vi "StitchAxialZones.vi"(4 "z increment axial":dbl=0.125, 5 "FileStartName":string, 6 "pressures in":dbl[][][](array[numeric]), 7 "Scales":dbl[](array[numeric]), 8 "z increment":dbl=0.125, 9 "z Start pos":sgl=7.0) -> (0 "6dB data":dbl[][](array[numeric]), 1 "Focal zones joined":dbl[][](array[numeric]), 2 "Axial Beam":cluster{sgl, dbl, sgl[]}(graph), 3 "lateral segs":cluster{dbl, dbl, dbl[][]}(graph))   [LabVIEW 2022 SP3]
uses:
  <vilib>/Math Plots/3D Math Plots/3D Surface/3D Surface XCtrl/3D Surface.xctl
  <vilib>/Math Plots/3D Math Plots/3D Surface/3D Surface Datatype/Public/Plot Helper (Vector).vi
  <vilib>/Utility/file.llb/Write Delimited Spreadsheet (DBL).vi
  <vilib>/Math Plots/3D Math Plots/3D Surface/3D Surface Datatype/3D Surface Datatype.lvclass
panel:
  in  "Tab Control":enum32{"Page 1", "Page 2"}(tab)
  out "Lateral 6dB":cluster{dbl[], dbl[]}(graph)
  out "Axia focal zone stitch":cluster{dbl[], dbl[]}(graph)
  in  "Save lateal profiles":bool
  in  "Save lateal BWs":bool
  in  "Save axial profile":bool
  out "3D Surface":refnum<class "3D Plot Datatype.lvclass">[](xcontrol)
  out "axial segs":cluster{sgl, dbl, dbl[][]}(graph)
  in  "Folder to place saved data":path=path "D:/"
  in  "P(t) or I(f)":bool
  out "max index(es)":i32[](array[numeric])
  out "dimension":i32[](array[numeric])
  out "step size":dbl
  out "subarray":dbl[][](array[numeric])
  # "Index 1 for lateral\nIndex 2 for axial"
  # "Focal zone only calc"
  # "Full beam sims axial assembly"
  # "Rerun just this VI and press buttons to save data in each plot"
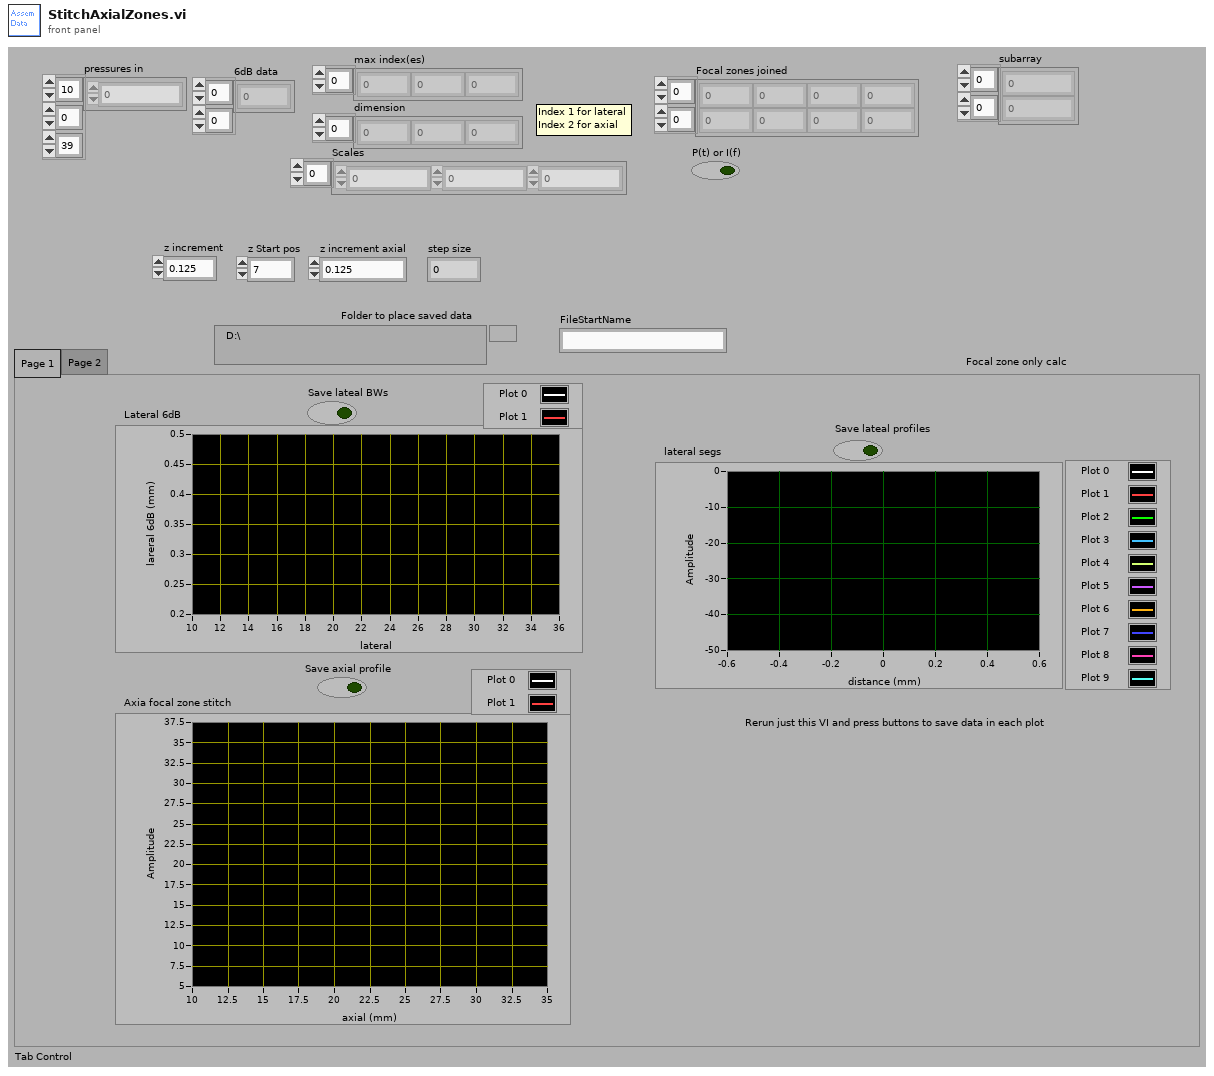
[diagram p1: front panel]
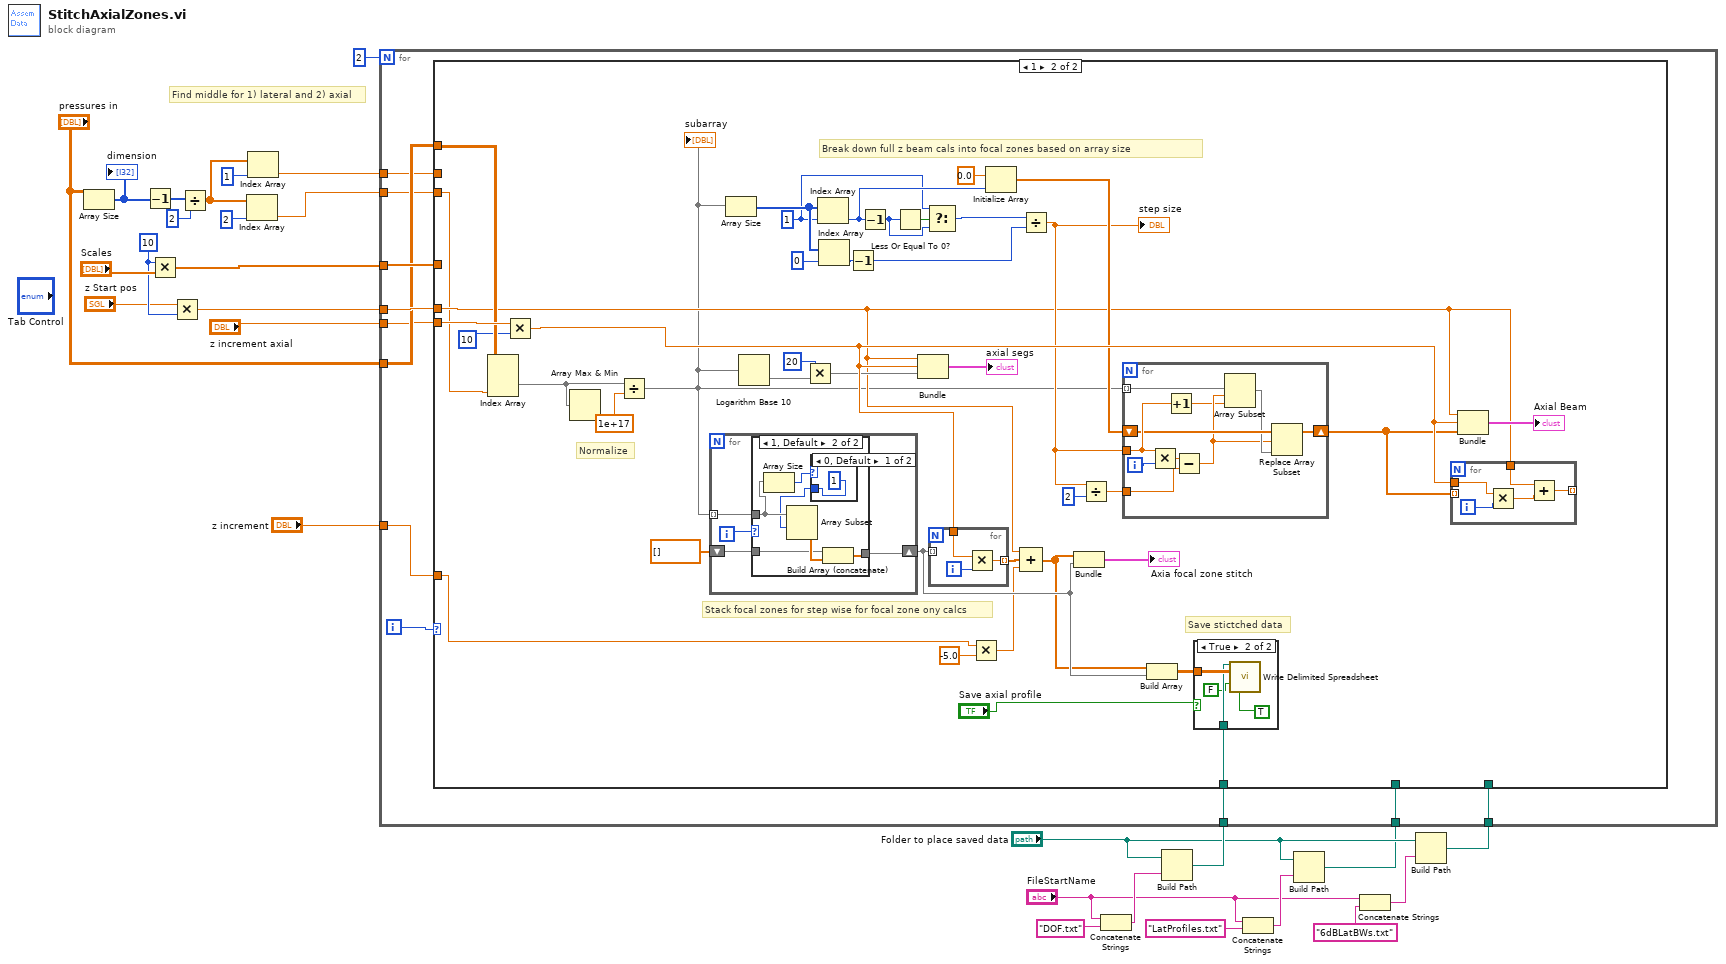
[diagram p0: block diagram]
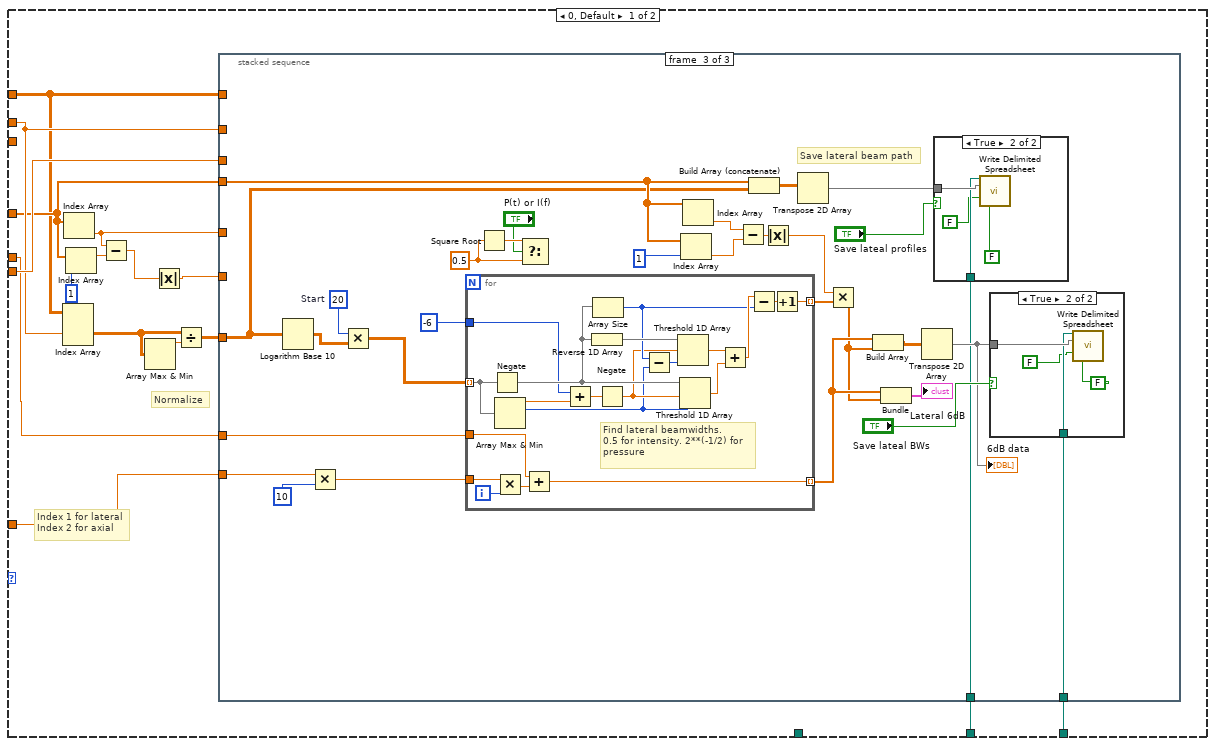
[diagram p2: hidden frame]
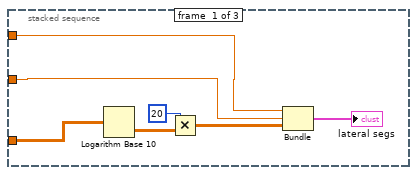
[diagram p3: hidden frame]
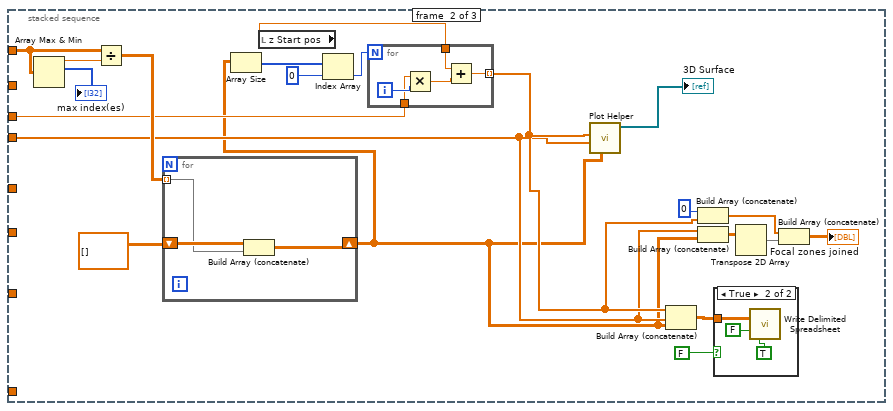
[diagram p4: hidden frame]
diagram:
  w25 = 10
  # "Find middle for 1) lateral and 2) axial"
  n1 = Array Size(array="pressures in") -> (size(s)=w18:i32[])
  "dimension" <- w18
  n2 = Decrement(x=w18) -> (x-1=w17:i32[])
  n3 = Multiply(x=w25, y="Scales") -> (x*y=w26:dbl[])
  n4 = Multiply(x="z Start pos", y=w25) -> (x*y=w23:sgl)
  n5 = Divide(x=w17, y=2) -> (x/y=w13:dbl[])
  n6 = Index Array(array=w13, index=2) -> (element=w15:dbl)
  n7 = Index Array(array=w13, index=1) -> (element=w12:dbl)
  n8 = Concatenate Strings("FileStartName", "DOF.txt") -> (w6:string)
  n9 = Build Path(base path="Folder to place saved data", name or relative path=w6) -> (appended path=w10:path)
  n10 = Concatenate Strings("FileStartName", "LatProfiles.txt") -> (w4:string)
  n11 = Build Path(base path="Folder to place saved data", name or relative path=w4) -> (appended path=w8:path)
  n12 = Concatenate Strings("FileStartName", "6dBLatBWs.txt") -> (w1:string)
  n13 = Build Path(base path="Folder to place saved data", name or relative path=w1) -> (appended path=w11:path)
  n14 = for {
    N: 2 -> [_]
    tunnel: "pressures in" -> [w37]
    tunnel: w26 -> [w39]
    tunnel: w23 -> [w38]
    tunnel: "z increment axial" -> [w34]
    tunnel: "z increment" -> [w35]
    tunnel: w15 -> [w33]
    tunnel: w12 -> [w32]
    tunnel: w11 -> [w31]
    tunnel: w10 -> [w30]
    tunnel: w8 -> [w29]
    i -> [w36]
    n15 = case shown="1" w36 {
      tunnel: w39 -> [w43 _]
      tunnel: w38 -> [w44 w160]
      tunnel: w34 -> [w50 w191]
      tunnel: w37 -> [w41 w190]
      tunnel: w35 -> [w46 w153]
      tunnel: w33 -> [_ w154]
      tunnel: w32 -> [w45 _]
      tunnel: w31 -> [w42 _]
      tunnel: w30 -> [_ w163]
      tunnel: w29 -> [w40 _]
      frame 0, Default {
        # "Normalize"
        # "Index 1 for lateral\nIndex 2 for axial"
        n16 = Index Array(array=w41, index (dim 1)=w45) -> (element=w54:dbl[][])  [unwired: 2 in]
        n17 = Index Array(array=w43) -> (element=w51:dbl)  [unwired: 1 in]
        n18 = Index Array(array=w43, index=1) -> (element=w49:dbl)
        n19 = Subtract(x=w51, y=w49) -> (x-y=w48:dbl)
        n20 = Array Max & Min(array=w54) -> (max value=w55:dbl)  [unwired: 3 out]
        n21 = Absolute Value(x=w48) -> (abs(x)=w52:dbl)
        n22 = Divide(x=w54, y=w55) -> (x/y=w53:dbl[][])
        n23 = stacked-sequence {
          tunnel: w53 -> [w59 _ w101]
          tunnel: w52 -> [w61 _ _]
          tunnel: w51 -> [w60 _ _]
          tunnel: w43 -> [_ w64 w112]
          tunnel: w41 -> [_ w80 _]
          tunnel: w44 -> [_ _ w111]
          tunnel: w46 -> [_ _ w107]
          tunnel: w50 -> [_ w73 _]
          tunnel: w45 -> [_ _ _]
          tunnel: w42 -> [_ _ w96]
          tunnel: w40 -> [_ _ w95]
          frame #0 {
            n24 = Logarithm Base 10(1:w59) -> (0:w57:dbl[][])
            n25 = Multiply(x=20, y=w57) -> (x*y=w56:dbl[][])
            n26 = Bundle(w60, w61, w56) -> (→"lateral segs":cluster{dbl, dbl, dbl[][]})  [unwired: 1 out]
          }
          frame #1 {
            n27 = Array Max & Min(array=w80) -> (max value=w82:dbl, max index (indices)=→"max index(es)":i32[])  [unwired: 2 out]
            n28 = Divide(x=w80, y=w82) -> (x/y=w77:dbl[][][])
            n29 = for {
              tunnel: w77 -> [w92] mode=indexing
              shift-right: [w94] -> w63
              shift-left: dbl[][] [] ("New Value") -> [w93]
              n30 = Build Array (concatenate)(w93, w92) -> (w94:dbl[][])
            }
            n31 = Array Size(array=w63) -> (size(s)=w76:i32[])
            n32 = local read "z Start pos"() -> (w72:sgl)
            n33 = Index Array(array=w76, index=0) -> (element=w74:i32)
            n34 = for {
              N: w74 -> [_]
              tunnel: [w86] -> w65 mode=indexing
              tunnel: w73 -> [w85]
              tunnel: w72 -> [w84]
              i -> [w88]
              n35 = Multiply(x=w85, y=w88) -> (x*y=w87:dbl)
              n36 = Add(x=w84, y=w87) -> (x+y=w86:dbl)
            }
            n37 = call-poly <vilib>:"Plot Helper.vi"("z matrix"=w63, "y vector"=w64, "x vector"=w65) -> ("3D Plot lvclass Array out"=→"3D Surface":refnum<class "3D Plot Datatype.lvclass">[])  [unwired: 3 in, 5 out]
            n38 = Build Array (concatenate)(w65, w64, w63) -> (w79:dbl[][])
            n39 = Build Array (concatenate)(0, w65) -> (w70:dbl[])
            n40 = Build Array (concatenate)(w64, w63) -> (w71:dbl[][])
            n41 = case shown="True" FALSE ("Case Constant\n(See Context Help)") {
              tunnel: w79 -> [_ w91]
              frame False {
              }
              frame True {
                n42 = call-poly <vilib>:"Write Delimited Spreadsheet.vi"("2D data"=w91, "append to file? (new file:F)"=FALSE, "transpose? (no:F)"=TRUE) -> ()  [unwired: 11 in, 2 out]
              }
            }
            n43 = Transpose 2D Array(2D array=w71) -> (transposed array=w69:dbl[][])
            n44 = Build Array (concatenate)(w70, w69) -> (→"Focal zones joined":dbl[][])
          }
          frame #2 {
            w105 = 0.5
            w99 = 20  # Start
            # "Save lateral beam path"
            n45 = Logarithm Base 10(1:w101) -> (0:w100:dbl[][])
            n46 = Multiply(x=w107, y=10) -> (x*y=w106:dbl)
            n47 = Multiply(x=w99, y=w100) -> (x*y=w98:dbl[][])
            n48 = for {
              tunnel: w98 -> [w132] mode=indexing
              tunnel: [w138] -> w116 mode=indexing
              tunnel: w106 -> [w136]
              tunnel: w111 -> [w134]
              tunnel: [w133] -> w120 mode=indexing
              tunnel: -6 -> [w129]
              i -> [w137]
              # "Find lateral beamwidths.\n0.5 for intensity. 2**(-1/2) for\npressure"
              n49 = Negate(x=w132) -> (-x=w141:dbl[])
              n50 = Array Max & Min(array=w132) -> (max value=w131:dbl, max index (indices)=w130:i32)  [unwired: 2 out]
              n51 = Multiply(x=w136, y=w137) -> (x*y=w135:dbl)
              n52 = Add(x=w134, y=w135) -> (x+y=w133:dbl)
              n53 = Add(x=w129, y=w131) -> (x+y=w145:dbl)
              n54 = Reverse 1D Array(array=w141) -> (reversed array=w148:dbl[])
              n55 = Array Size(array=w141) -> (size(s)=w142:i32)
              n56 = Negate(x=w145) -> (-x=w140:dbl)
              n57 = Subtract(x=w142, y=w130) -> (x-y=w144:i32)
              n58 = Threshold 1D Array(1:w144, 2:w140, 3:w148) -> (0:w147:dbl)
              n59 = Threshold 1D Array(1:w130, 2:w140, 3:w141) -> (0:w146:dbl)
              n60 = Add(x=w147, y=w146) -> (x+y=w143:dbl)
              n61 = Subtract(x=w143, y=w142) -> (x-y=w139:dbl)
              n62 = Increment(x=w139) -> (x+1=w138:dbl)
            }
            n63 = Square Root(x=w105) -> (sqrt(x)=w104:dbl)
            n64 = Select(t=w104, s="P(t) or I(f)", f=w105) -> ()  [unwired: 1 out]
            n65 = Index Array(array=w112, index=1) -> (element=w123:dbl)
            n66 = Index Array(array=w112) -> (element=w122:dbl)  [unwired: 1 in]
            n67 = Subtract(x=w122, y=w123) -> (x-y=w115:dbl)
            n68 = Build Array (concatenate)(w112, w101) -> (w124:dbl[][])
            n69 = Absolute Value(x=w115) -> (abs(x)=w121:dbl)
            n70 = Transpose 2D Array(2D array=w124) -> (transposed array=w113:dbl[][])
            n71 = Multiply(x=w121, y=w116) -> (x*y=w117:dbl[])
            n72 = Build Array(w120, w117) -> (w119:dbl[][])
            n73 = Bundle(w120, w117) -> (→"Lateral 6dB":cluster{dbl[], dbl[]})  [unwired: 1 out]
            n74 = Transpose 2D Array(2D array=w119) -> (transposed array=w102:dbl[][])
            "6dB data" <- w102
            n75 = case shown="True" "Save lateal profiles" {
              tunnel: w113 -> [_ w151]
              tunnel: w95 -> [_ w150]
              frame False {
              }
              frame True {
                n76 = call-poly <vilib>:"Write Delimited Spreadsheet.vi"("file path (dialog if empty)"=w150, "2D data"=w151, "append to file? (new file:F)"=FALSE, "transpose? (no:F)"=FALSE) -> ()  [unwired: 10 in, 2 out]
              }
            }
            n77 = case shown="True" "Save lateal BWs" {
              tunnel: w102 -> [_ w128]
              tunnel: w96 -> [_ w127]
              frame False {
              }
              frame True {
                n78 = call-poly <vilib>:"Write Delimited Spreadsheet.vi"("file path (dialog if empty)"=w127, "2D data"=w128, "append to file? (new file:F)"=FALSE, "transpose? (no:F)"=FALSE ("append to file? (new file:F)")) -> ()  [unwired: 10 in, 2 out]
              }
            }
          }
        }
      }
      frame 1 {
        w172 = 1
        # "Save stictched data"
        # "Stack focal zones for step wise for focal zone ony calcs"
        # "Break down full z beam cals into focal zones based on array size"
        # "Normalize"
        n79 = Index Array(array=w190, index (dim 2)=w154) -> (element=w159:dbl[][])  [unwired: 2 in]
        n80 = Multiply(x=w191, y=10) -> (x*y=w192:dbl)
        n81 = Array Max & Min(array=w159) -> ()  [unwired: 4 out]
        n82 = Divide(x=w159, y=1e+17 ("max value")) -> (x/y=w158:dbl[][])
        "subarray" <- w158
        n83 = for {
          tunnel: w158 -> [w201] mode=indexing
          shift-right: [w202] -> w177
          shift-left: dbl[] [] -> [w203]
          i -> [w200]
          n84 = case shown="1, Default" w200 {
            tunnel: w203 -> [_ w208]
            tunnel: [w204 w210] -> w202
            tunnel: w201 -> [w204 w207]
            frame 0 {
            }
            frame 1, Default {
              n85 = Array Size(array=w207) -> (size(s)=w206:i32)
              n86 = case shown="0, Default" w206 {
                tunnel: [1 _] -> w205
                frame 0, Default {
                }
                frame 1 {
                }
              }
              n87 = Array Subset(array=w207, index=w205) -> (w209:dbl[])  [unwired: 1 in]
              n88 = Build Array (concatenate)(w208, w209) -> (w210:dbl[])
            }
          }
        }
        n89 = Array Size(array=w158) -> (size(s)=w188:i32[])
        n90 = Logarithm Base 10(1:w158) -> (0:w175:dbl[][])
        n91 = Multiply(x=20, y=w175) -> (x*y=w174:dbl[][])
        n92 = Index Array(array=w188, index=w172) -> (element=w179:i32)
        n93 = Index Array(array=w188, index=0) -> (element=w186:i32)
        n94 = Decrement(x=w186) -> (x-1=w185:i32)
        n95 = Decrement(x=w179) -> (x-1=w171:i32)
        n96 = Less Or Equal To 0?(x=w171) -> (x <= 0?=w173:bool)
        n97 = Bundle(w160, w192, w174) -> (→"axial segs":cluster{sgl, dbl, dbl[][]})  [unwired: 1 out]
        n98 = Select(t=w172, s=w173, f=w171) -> (s? t:f=w170:i32)
        n99 = for {
          tunnel: w177 -> [_] mode=indexing
          tunnel: w192 -> [w198]
          tunnel: [w197] -> w162 mode=indexing
          i -> [w199]
          n100 = Multiply(x=w198, y=w199) -> (x*y=w197:dbl)
        }
        n101 = Multiply(x=w153, y=-5.0) -> (x*y=w155:dbl)
        n102 = Initialize Array(sgl 0.0, w179) -> (w183:sgl[])
        n103 = Compound Arithmetic op=ADD(w160, w162, w155) -> (w161:dbl[])
        n104 = Divide(x=w170, y=w185) -> (x/y=w165:dbl)
        "step size" <- w165
        n105 = Bundle(w161, w177) -> (→"Axia focal zone stitch":cluster{dbl[], dbl[]})  [unwired: 1 out]
        n106 = Divide(x=w165, y=2) -> (x/y=w180:dbl)
        n107 = for {
          tunnel: w165 -> [w224]
          tunnel: w158 -> [w226] mode=indexing
          shift-right: [w222] -> w182
          shift-left: w183 -> [w223]
          tunnel: w180 -> [w218]
          i -> [w225]
          n108 = Multiply(x=w224, y=w225) -> (x*y=w220:dbl)
          n109 = Increment(x=w224) -> (x+1=w217:dbl)
          n110 = Subtract(x=w220, y=w218) -> (x-y=w219:dbl)
          n111 = Array Subset(array=w226, index=w219, length=w217) -> (w221:dbl[])
          n112 = Replace Array Subset(array=w223, new element=w221, index=w219) -> (w222:sgl[])
        }
        n113 = Build Array(w161, w177) -> (w178:dbl[][])
        n114 = case shown="True" "Save axial profile" {
          tunnel: w178 -> [_ w196]
          tunnel: w163 -> [_ w195]
          frame False {
          }
          frame True {
            n115 = call-poly <vilib>:"Write Delimited Spreadsheet.vi"("file path (dialog if empty)"=w195, "2D data"=w196, "append to file? (new file:F)"=FALSE, "transpose? (no:F)"=TRUE) -> ()  [unwired: 10 in, 2 out]
          }
        }
        n116 = for {
          tunnel: w192 -> [w215]
          tunnel: w160 -> [w213]
          tunnel: [w212] -> _ mode=indexing
          tunnel: w182 -> [_] mode=indexing
          i -> [w216]
          n117 = Multiply(x=w215, y=w216) -> (x*y=w214:dbl)
          n118 = Add(x=w213, y=w214) -> (x+y=w212:dbl)
        }
        n119 = Bundle(w160, w192, w182) -> (→"Axial Beam":cluster{sgl, dbl, sgl[]})  [unwired: 1 out]
      }
    }
  }
